vi "w0 via 2nd mom 1D.vi"(7 "Threshold for 2nd mom":dbl=0.05 format="%#_13g", 10 "Input array":dbl[](graph), 11 "Centroid":sgl) -> (3 "w0 via 2nd mom":sgl)   [LabVIEW 2020]
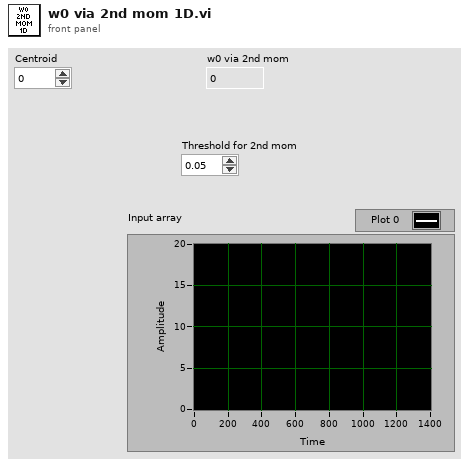
[diagram p1: front panel]
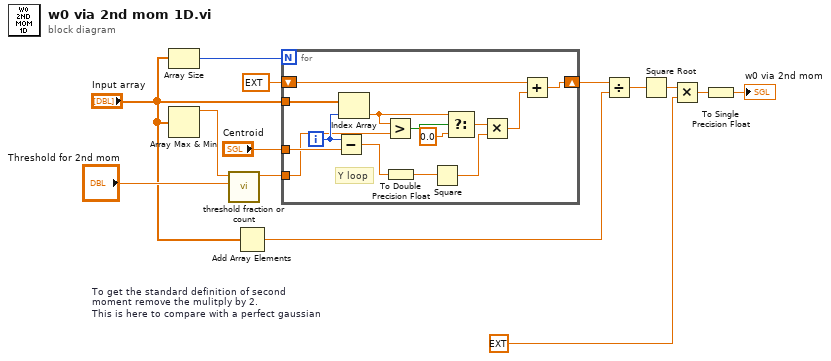
[diagram p0: block diagram]
diagram:
  w8 = ext 2.0  # To get the standard definition of second moment remove the mulitply by 2. This is here to compare with a perfect gaussian
  n1 = Array Size(array="Input array") -> (size(s)=w4:i32)
  n2 = Array Max & Min(array="Input array") -> (max value=w12:dbl)  [unwired: 3 out]
  n3 = call "threshold fraction or count.vi"("Threshold in"="Threshold for 2nd mom", "Maximal Value"=w12) -> ("Threshold out"=w14:dbl)  [unwired: 9 in]
  n4 = Add Array Elements(numeric array="Input array") -> (sum=w1:dbl)
  n5 = for {
    N: w4 -> [_]
    tunnel: "Input array" -> [w28]
    tunnel: "Centroid" -> [w26]
    shift-right: [w22] -> w9
    shift-left: ext 0.0 -> [w21]
    tunnel: w14 -> [w19]
    i -> [w27]
    # "Y loop"
    n6 = Subtract(x=w27, y=w26) -> (x-y=w25:sgl)
    n7 = Index Array(array=w28, index=w27) -> (element=w17:dbl)
    n8 = Greater?(x=w17, y=w19) -> (0:w18:bool)
    n9 = To Double Precision Float(number=w25) -> (double precision float=w20:dbl)
    n10 = Square(x=w20) -> (x^2=w24:dbl)
    n11 = Select(t=w17, s=w18, f=sgl 0.0) -> (s? t:f=w16:dbl)
    n12 = Multiply(x=w16, y=w24) -> (x*y=w23:dbl)
    n13 = Add(x=w21, y=w23) -> (x+y=w22:ext)
  }
  n14 = Divide(x=w9, y=w1) -> (x/y=w7:ext)
  n15 = Square Root(x=w7) -> (sqrt(x)=w6:ext)
  n16 = Multiply(x=w6, y=w8) -> (x*y=w10:ext)
  n17 = To Single Precision Float(number=w10) -> (single precision float=→"w0 via 2nd mom":sgl)
